vi "wfsettings.vi"(2 "error in":errorcluster, 3 "wfsettings in":T1, 4 "command":string="set") -> (0 "Error out":errorcluster, 1 "wfsettings out":T1)   [LabVIEW 2015]
panel:
  # "it's possible to manually add settings to this buffer. at the beginning of the program, it \nwill load your list into memory.\nmake sure that, when you add one manually, or via the program, that you select \"make current values default\"\nand save."
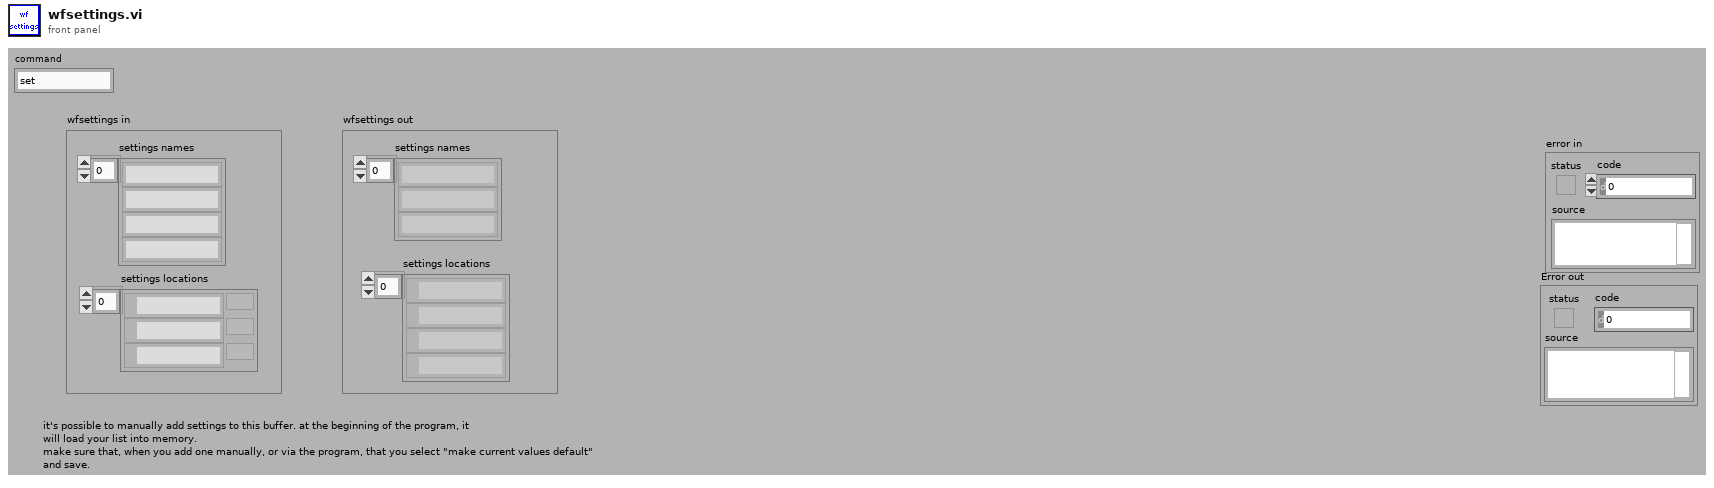
[diagram p1: front panel]
types:
  T1 = cluster{"settings names":string[], "settings locations":path[]}
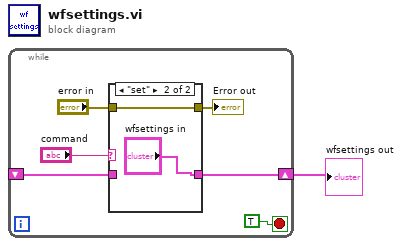
[diagram p0: block diagram]
diagram:
  n1 = while {
    shift-right: [w5] -> w1
    shift-left: _ -> [w4]
    stop <- TRUE stop-if-true
    n2 = case shown="\"set\"" "command" {
      tunnel: [w9 "wfsettings in"] -> w5
      tunnel: w4 -> [w9 _]
      tunnel: [w8 w11] -> w3
      tunnel: "error in" -> [w8 w11]
      frame "get", Default {
      }
      frame "set" {
      }
    }
    "Error out" <- w3
  }
  "wfsettings out" <- w1
